vi "Config - CheckIfStable.vi"(8 "Fehler (Eingang, kein Fehler)":errorcluster) -> (0 "Fehler (Ausgang)":errorcluster)   [LabVIEW 2016]
uses:
  eGateUtility.dll
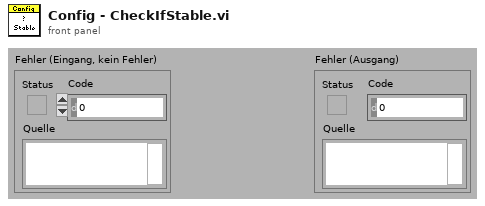
[diagram p1: front panel]
types:
  T1 = enum16{"open", "replace", "create", "open or create", "replace or create", "replace or create with confirmation"}
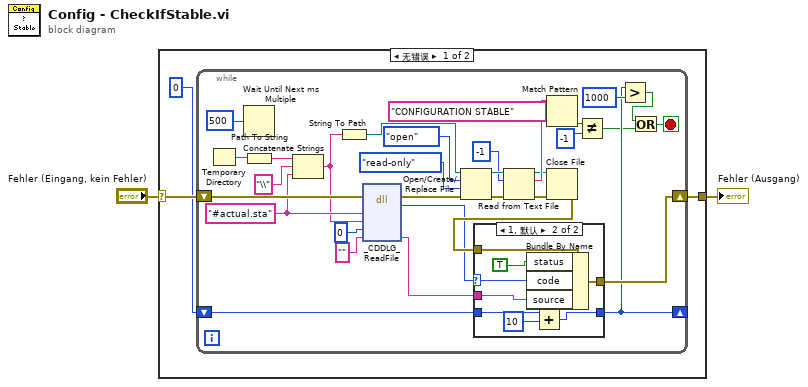
[diagram p0: block diagram]
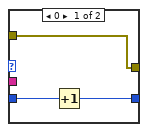
[diagram p2: hidden frame]
diagram:
  n1 = case shown="无错误" "Fehler (Eingang, kein Fehler)" {
    selector: "Fehler (Eingang, kein Fehler)" -> [w4 w49]
    tunnel: [w5 w49] -> w2
    frame No Error {
      n2 = while {
        shift-right: [w14] -> w5
        shift-left: w4 -> [w37]
        shift-right: [w9] -> _
        shift-left: 0 -> [w10]
        stop <- w8 stop-if-true
        w36 = "#actual.sta" ("SourceFileName")
        n3 = Temporary Directory() -> (w17:path)
        n4 = Wait Until Next ms Multiple(millisecond multiple=u32 500 ("Vielfache von ms")) -> ()  [unwired: 1 out]
        n5 = Path To String(path=w17) -> (string=w16:string)
        n6 = Concatenate Strings(w16, "\\" ("String"), w36) -> (w31:string)
        n7 = String To Path(string=w31) -> (path=w30:path)
        n8 = dll-call lib="eGateUtility.dll" fn="_CDDLG_ReadFile"(error in=w37, "SourceFileName"=w36, "DestinationFullFileName"=w31, "AppendToExisting"=0, "ErrorString"="") -> (error out=w32:errorcluster, "Rückgabetyp"=w12:i32, "ErrorString"=w13:string)  [unwired: 4 in, 2 out]
        n9 = Open/Create/Replace File(file path (use dialog)=w30, error in=w32, operation (0:open)=T1."open" ("Operation (0:Öffnen)"), access (0:read/write)=enum16{"read/write", "read-only", "write-only"}."read-only" ("Zugriff (0:Lesen/Schreiben)")) -> (refnum out=w27:refnum<file>, error out=w26:errorcluster)  [unwired: 3 out]
        n10 = Read from Text File(file (use dialog)=w27, count=-1 ("Anzahl"), error in=w26) -> (refnum out=w18:refnum<file>, text=w23:string, error out=w19:errorcluster)  [unwired: 2 out]
        n11 = Match Pattern(string=w23, regular expression="CONFIGURATION STABLE" ("Regulärer Ausdruck")) -> (offset past match=w21:i32)  [unwired: 4 out]
        n12 = Close File(refnum=w18, error in=w19) -> (error out=w15:errorcluster)  [unwired: 1 out]
        n13 = case shown="1, 默认" w12 {
          selector: w12 -> [_ w45]
          tunnel: w15 -> [w40 w48]
          tunnel: [w40 w47] -> w14
          tunnel: w13 -> [_ w46]
          tunnel: w10 -> [w39 w43]
          tunnel: [w38 w42] -> w9
          frame 0 {
            n14 = Increment(x=w39) -> (x+1=w38:i32)
          }
          frame 1, Default {
            n15 = Bundle By Name(cluster=w48, "status"=TRUE, "code"=w45, "source"=w46) -> (w47:errorcluster)
            n16 = Add(x=w43, y=10) -> (x+y=w42:i32)
          }
        }
        n17 = Not Equal?(x=w21, y=-1) -> (x != y?=w7:bool)
        n18 = Greater?(x=w9, y=1000) -> (0:w6:bool)
        n19 = Or(x=w6, y=w7) -> (x .or. y?=w8:bool)
      }
    }
    frame Error {
    }
  }
  "Fehler (Ausgang)" <- w2
